vi "Write Legend Plot Visibility.vi"(5 "Legend Plot Visibility":bool, 9 "WaveformChart in":refnum<class "WaveformGraph.lvclass">) -> (3 "WaveformChart out":refnum<class "WaveformGraph.lvclass">)   [LabVIEW 2014, in "Raspberry Pi Compatible Compiler for LabVIEW.lvlib" / "WaveformGraph.lvclass"]
uses:
  WaveformGraph.lvclass
  WaveformGraph.lvclass/WaveformGraph.ctl
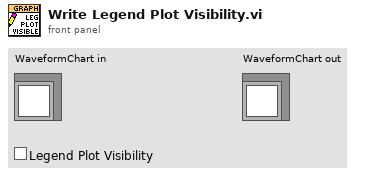
[diagram p1: front panel]
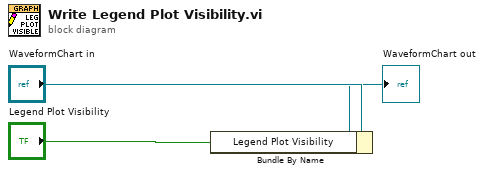
[diagram p0: block diagram]
diagram:
  n1 = Bundle By Name(cluster="WaveformChart in", "Legend Plot Visibility"="Legend Plot Visibility") -> (→"WaveformChart out":refnum<class "WaveformGraph.lvclass">)
